vi "avaliaGoleiroForaArea.vi"(10 "Robot in":T1, 11 "IA State":T6={"our_robots"=[], "enemy_robots"=[], "balls"=[], "geometry"={"field_length"=0, "field_width"=0, "goal_width"=0, "goal_depth"=0, "center_circle_radius"=0, "defense_width"=0, "defense_depth"=0, "free_kick_from_defense_dist"=0, "penalty_spot_from_field_line_dist"=0, "penalty_line_from_spot_dist"=0, "half_moon_depth"=0, "half_moon_width"=0}, "IA Judge"={"stage"="", "command"="", "our_goalie_id"=0.0, "enemy_goalie_id"=0.0, "command enum"=enum."Halt", "Time"=enum."Azul"}, "Received Timestamp"=timestamp(0 s since 1904-01-01), "Events"={"Touch"=FALSE, "id touch"=0.0, "Ball out of \nVision"=FALSE, "Ball inside \nGoalie area"=FALSE, "Robot not responding"=FALSE, "Robots responding status"=[1.0, 1.0, 1.0, 1.0, 1.0, 1.0], "Enemy Ball \nPossession"=FALSE, "Id ini Possession"=0.0, "Ball Possesion"=FALSE, "Id Possesion"=0.0, "Ball at\nour goal side"=FALSE, "Ball at\ntouchline"=FALSE, "Ball at\nenemy goal side"=FALSE}}) -> (3 "Goleiro fora da área?":bool=TRUE)   [LabVIEW 2018]
doc: "Função que avalia se o Goleiro está foraa da área."
uses:
  Core/AI Input.ctl
  Core/AI Robot.ctl
  Intel/Functions Enum.ctl
  Intel/AttackerStates.ctl
  Path Planning/RRT/PathDests.ctl
  Path Planning/RRT/PathDest.ctl
  Core/AI Ball.ctl
  Core/Field Size.ctl
  Core/AI Judge.ctl
  Intel/Command Enum.ctl
  Util/Events/Events.ctl
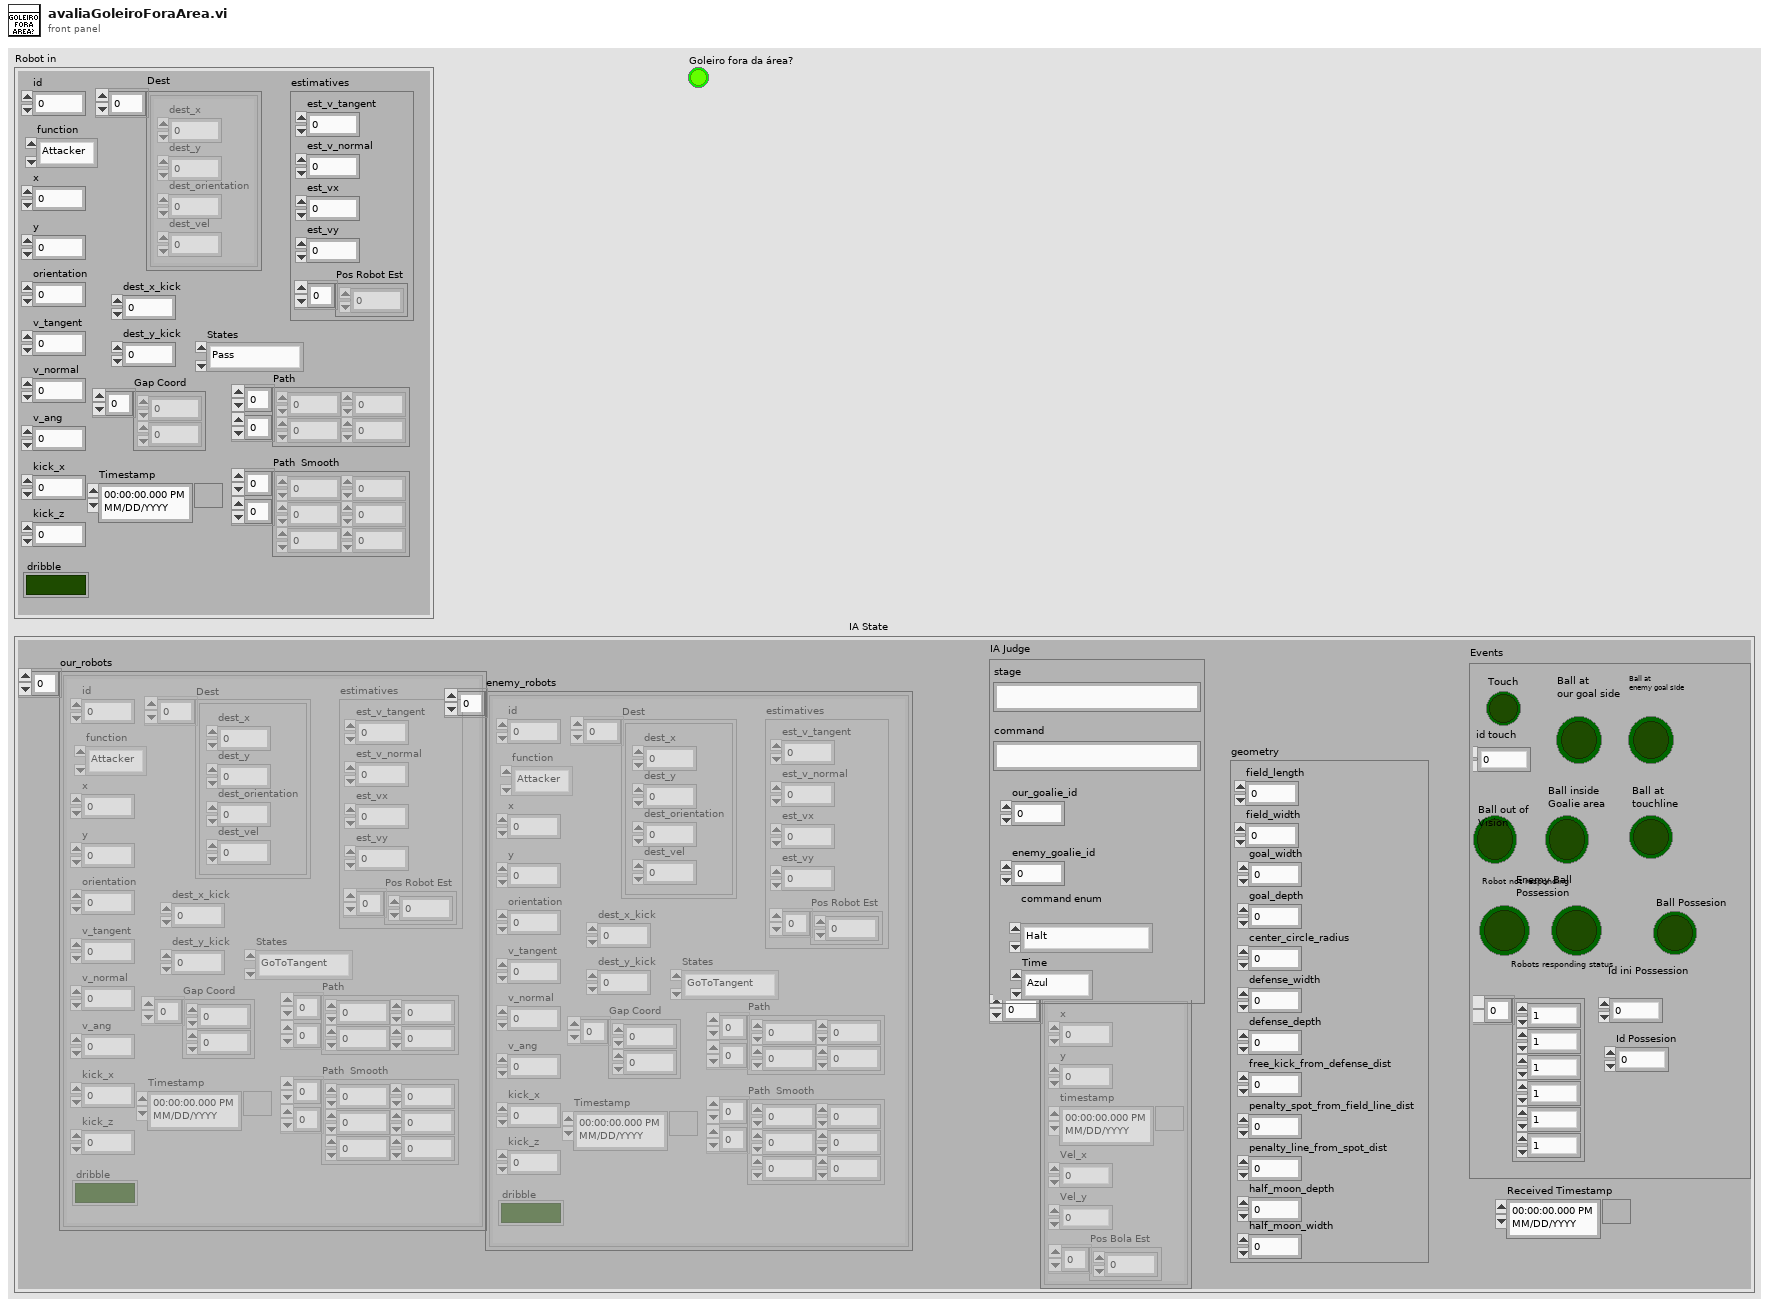
[diagram p1: front panel]
types:
  T1 = typedef "AI Robot.ctl" = cluster{"id":u32, "function":T2, "x":dbl, "y":dbl, "orientation":dbl, "v_tangent":dbl, "v_normal":dbl, "v_ang":dbl, "kick_x":dbl, "kick_z":dbl, "dribble":bool, "Timestamp":timestamp, "estimatives":cluster{"est_v_tangent":dbl, "est_v_normal":dbl, "est_vx":dbl, "est_vy":dbl, "Pos Robot Est":dbl[]}, "dest_x_kick":dbl, "dest_y_kick":dbl, "Gap Coord":dbl[], "States":T3, "Path ":dbl[][], "Path  Smooth":dbl[][], "Dest":T4}
  T2 = typedef "Functions Enum.ctl" = enum16{"Attacker", "Goalie", "Defender", "Striker", "Goto 0", "Dummy", "Kicker", "ZigZag"}
  T3 = typedef "AttackerStates.ctl" = enum16{"Pass", "GoToTangent", "BallGetting", "GoToKick", "Rotate anti-clockwise", "Rotate Clockwise", ""}
  T4 = typedef "PathDests.ctl" = T5[]
  T5 = typedef "PathDest.ctl" = cluster{"dest_x":dbl, "dest_y":dbl, "dest_orientation":dbl, "dest_vel":dbl}
  T6 = typedef "AI Input.ctl" = cluster{"our_robots":T1[], "enemy_robots":T1[], "balls":T7[], "geometry":T8, "IA Judge":T9, "Received Timestamp":timestamp, "Events":T11}
  T7 = typedef "AI Ball.ctl" = cluster{"x":dbl, "y":dbl, "timestamp":timestamp, "Vel_x":dbl, "Vel_y":dbl, "Pos Bola Est":dbl[]}
  T8 = typedef "Field Size.ctl" = cluster{"field_length":u32, "field_width":u32, "goal_width":u32, "goal_depth":u32, "center_circle_radius":u32, "defense_width":u32, "defense_depth":u32, "free_kick_from_defense_dist":u32, "penalty_spot_from_field_line_dist":u32, "penalty_line_from_spot_dist":u32, "half_moon_depth":u32, "half_moon_width":u32}
  T9 = typedef "AI Judge.ctl" = cluster{"stage":string, "command":string, "our_goalie_id":dbl, "enemy_goalie_id":dbl, "command enum":T10, "Time":enum16{"Azul", "Amarelo"}}
  T10 = typedef "Command Enum.ctl" = enum16{"Halt", "Stop", "Force Start", "PKA Normal Start", "Prepare Kickoff Ally", "PKE Normal Start", "Prepare Kickoff Enemy", "Prepare Penalty Ally", "PPA Normal Start", "Prepare Penalty Enemy", "PPE Normal Start", "Ball Placement Enemy Up", "Ball Placement Enemy Down", "Ball Placement Ally Up", "Ball Placement Ally Mid", "Ball Placement Ally Down", "Indirect Free Enemy", "Indirect Free Ally", "Timeout Enemy", "Timeout Ally", "Goal Enemy", "Goal Ally", "Normal Half Time", "Extra Time Break", "Extra Half Time", "None", "Post Game"}
  T11 = typedef "Events.ctl" = cluster{"Touch":bool, "id touch":dbl, "Ball out of \nVision":bool, "Ball inside \nGoalie area":bool, "Robot not responding":bool, "Robots responding status":dbl[], "Enemy Ball \nPossession":bool, "Id ini Possession":dbl, "Ball Possesion":bool, "Id Possesion":dbl, "Ball at\nour goal side":bool, "Ball at\ntouchline":bool, "Ball at\nenemy goal side":bool}
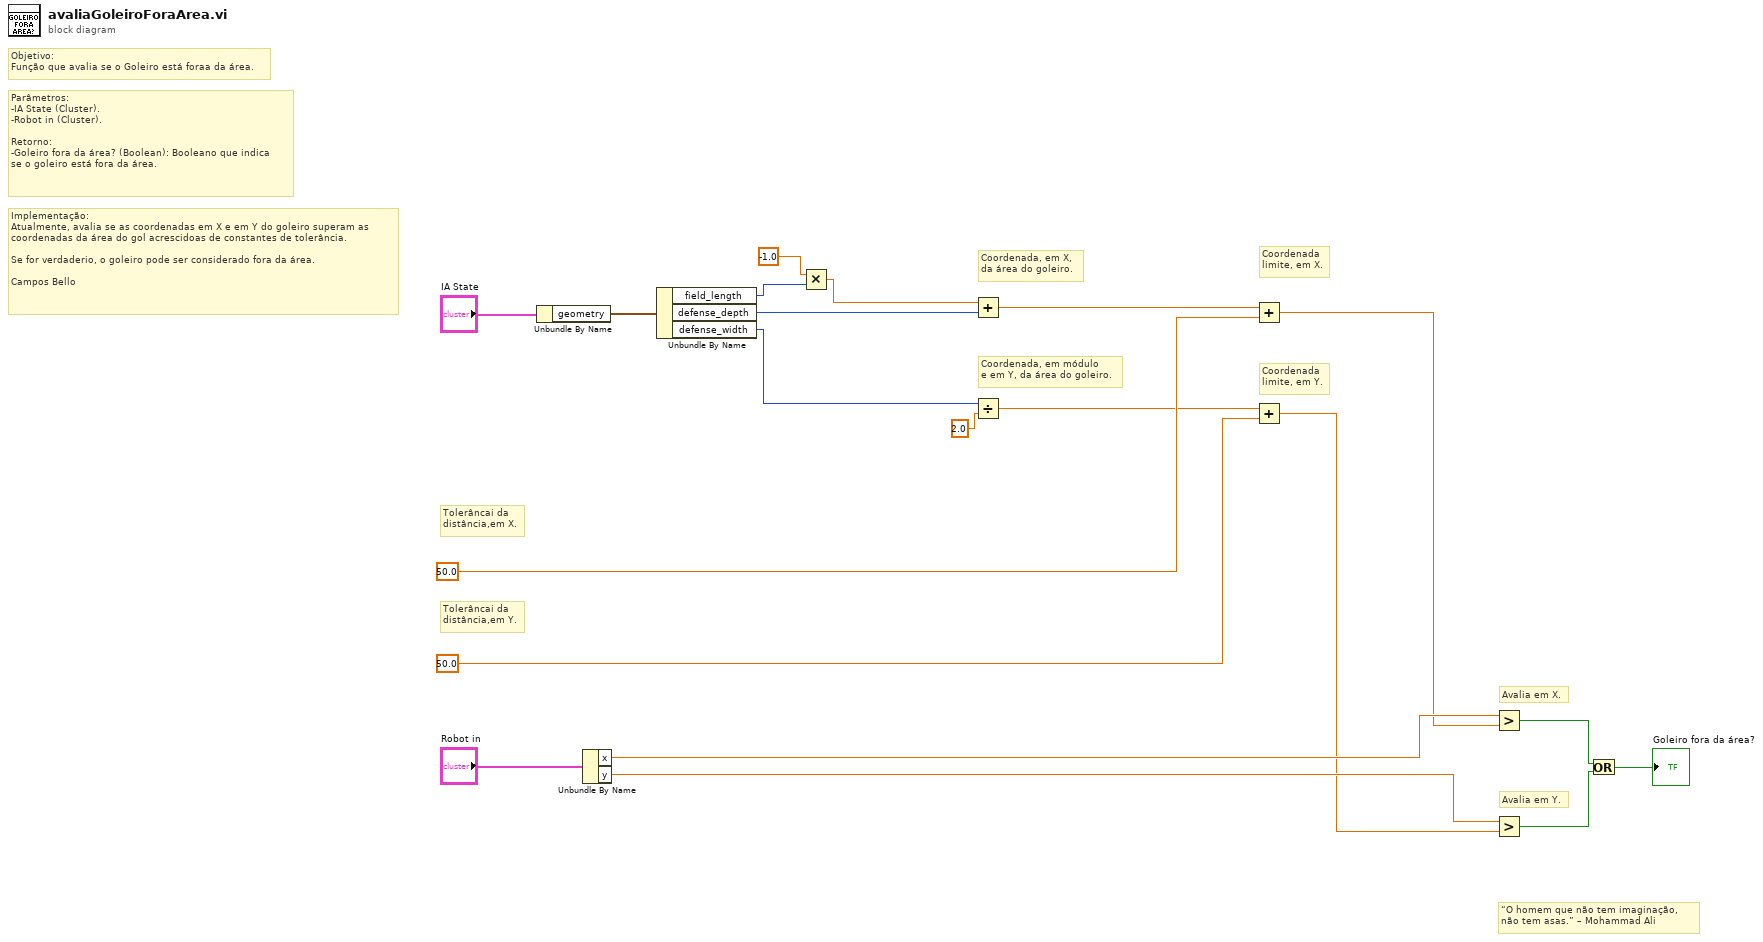
[diagram p0: block diagram]
diagram:
  # "“O homem que não tem imaginação,\nnão tem asas.” – Mohammad Ali"
  # "Implementação:\nAtualmente, avalia se as coordenadas em X e em Y do goleiro superam as\ncoordenadas da área do gol acrescidoas de constantes de tolerância.\n\nSe for verdaderio, o goleiro pode ser considerado fora da área.\n\nCampos Bello"
  # "Parâmetros:\n-IA State (Cluster).\n-Robot in (Cluster).\n\nRetorno:\n-Goleiro fora da área? (Boolean): Booleano que indica\nse o goleiro está fora da área."
  # "Objetivo:\nFunção que avalia se o Goleiro está foraa da área."
  # "Avalia em Y."
  # "Avalia em X."
  # "Coordenada\nlimite, em Y."
  # "Coordenada\nlimite, em X."
  # "Tolerâncai da\ndistância,em Y."
  # "Tolerâncai da\ndistância,em X."
  # "Coordenada, em módulo\ne em Y, da área do goleiro."
  # "Coordenada, em X,\nda área do goleiro."
  n1 = Unbundle By Name("IA State") -> ("geometry"=w19:T8)
  n2 = Unbundle By Name("Robot in") -> ("x"=w7:dbl, "y"=w6:dbl)
  n3 = Unbundle By Name(w19) -> ("field_length"=w17:u32, "defense_depth"=w15:u32, "defense_width"=w14:u32)
  n4 = Multiply(x=-1.0, y=w17) -> (x*y=w16:dbl)
  n5 = Add(x=w16, y=w15) -> (x+y=w10:dbl)
  n6 = Divide(x=w14, y=2.0 ("x/y")) -> (x/y=w9:dbl)
  n7 = Add(x=w10, y=50.0) -> (x+y=w5:dbl)
  n8 = Add(x=w9, y=50.0) -> (x+y=w4:dbl)
  n9 = Greater?(x=w7, y=w5) -> (0:w3:bool)
  n10 = Greater?(x=w6, y=w4) -> (0:w2:bool)
  n11 = Or(x=w3, y=w2) -> (x .or. y?=→"Goleiro fora da área?":bool)
